vi "Swerve Sensors RefNum Set.vi"(10 "Swerve Sensors DevRef":T1, 11 "Swerve Sensors Name":string) -> ()   [LabVIEW 2014]
uses:
  Swerve Sensors DevRef.ctl
  <vilib>/Rock Robotics/WPI/AnalogChannel/WPI_AnalogChannelDevRef.ctl
  <vilib>/Rock Robotics/SystemInterfaces/Typedef/FPGA_TypedefAnalogModule.ctl
  <vilib>/Rock Robotics/SystemInterfaces/AI/FPGA_AIChannel.ctl
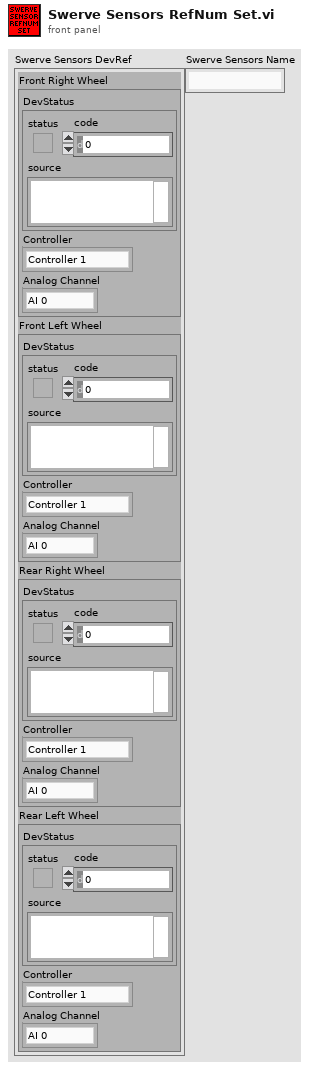
[diagram p1: front panel]
types:
  T1 = typedef "Swerve Sensors DevRef.ctl" = cluster{"Front Right Wheel":T2, "Front Left Wheel":T2, "Rear Right Wheel":T2, "Rear Left Wheel":T2}
  T2 = typedef "WPI_AnalogChannelDevRef.ctl" = cluster{"DevStatus":errorcluster, "Controller":T3, "Analog Channel":T4}
  T3 = typedef "FPGA_TypedefAnalogModule.ctl" = enum16{"Controller 1"}
  T4 = typedef "FPGA_AIChannel.ctl" = enum8{"AI 0", "AI 1", "AI 2", "AI 3", "AI MXP 0", "AI MXP 1", "AI MXP 2", "AI MXP 3", "Invalid"}
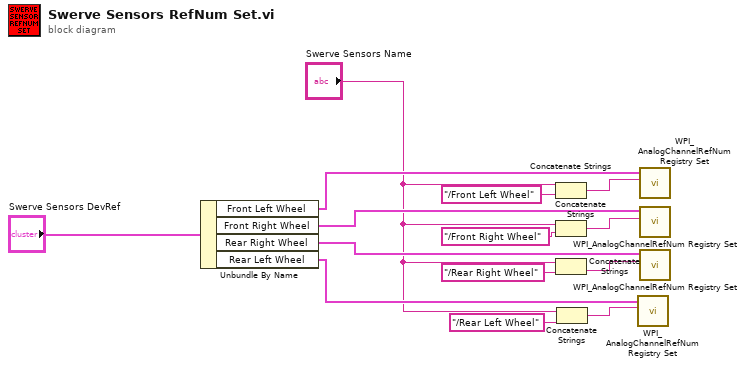
[diagram p0: block diagram]
diagram:
  n1 = Unbundle By Name("Swerve Sensors DevRef") -> ("Front Left Wheel"=w13:T2, "Front Right Wheel"=w6:T2, "Rear Right Wheel"=w11:T2, "Rear Left Wheel"=w10:T2)
  n2 = Concatenate Strings("Swerve Sensors Name", "/Front Left Wheel" ("string")) -> (w12:string)
  n3 = Concatenate Strings("Swerve Sensors Name", "/Front Right Wheel" ("string")) -> (w8:string)
  n4 = Concatenate Strings("Swerve Sensors Name", "/Rear Right Wheel" ("string")) -> (w7:string)
  n5 = Concatenate Strings("Swerve Sensors Name", "/Rear Left Wheel" ("string")) -> (w9:string)
  n6 = call <vilib>:"WPI_AnalogChannelRefNum Registry Set.vi"("refnum name"=w9, "AIDeviceRef"=w10) -> ()  [unwired: 8 in, 2 out]
  n7 = call <vilib>:"WPI_AnalogChannelRefNum Registry Set.vi"("refnum name"=w12, "AIDeviceRef"=w13) -> ()  [unwired: 8 in, 2 out]
  n8 = call <vilib>:"WPI_AnalogChannelRefNum Registry Set.vi"("refnum name"=w8, "AIDeviceRef"=w6) -> ()  [unwired: 8 in, 2 out]
  n9 = call <vilib>:"WPI_AnalogChannelRefNum Registry Set.vi"("refnum name"=w7, "AIDeviceRef"=w11) -> ()  [unwired: 8 in, 2 out]
